vi "Calculate Batch Offset Values.vi"(8 "error in":errorcluster, 9 "Site Data":T2[](array[typedef]), 10 "Cal Runtime Cfg":T5, 11 "Config Data":T4(array[cluster])) -> (0 "error out":errorcluster, 1 "Data String":string[][](array[string]), 2 "Col Header String":string[](array[string]), 3 "All Items Pass?":bool, 4 "Limit Status":T1)   [LabVIEW 2020, in "GUCalibration2.lvlib"]
uses:
  GUCalibration2.lvlib
  Controls/Config Data Type.ctl
  Controls/Site Data Element.ctl
  Controls/Site Raw Data Element.ctl
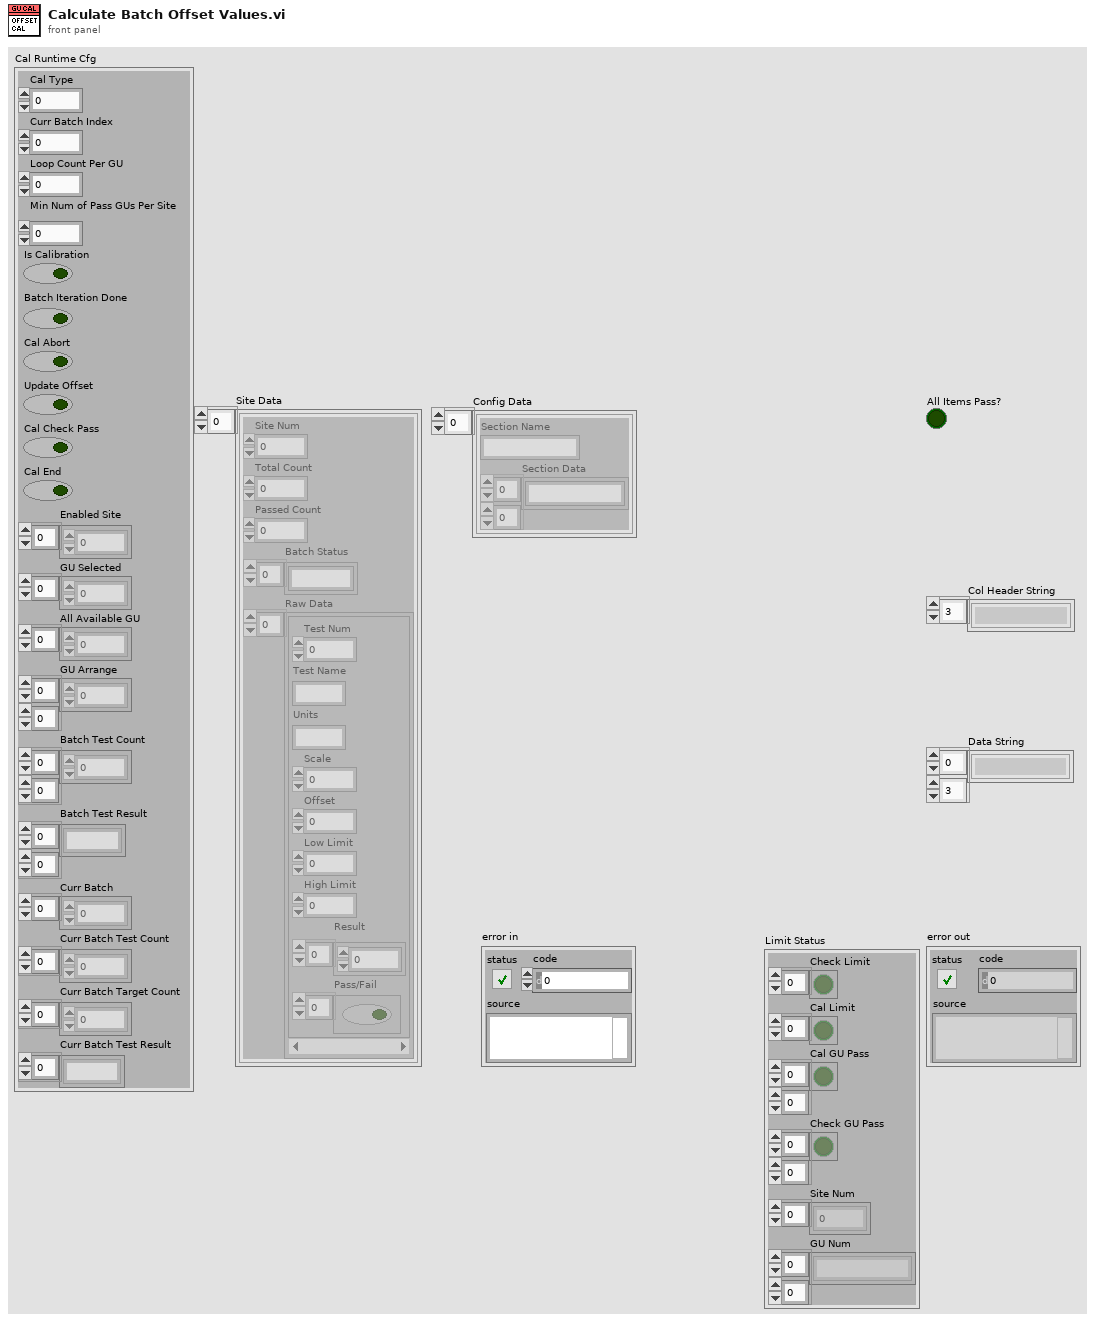
[diagram p1: front panel]
types:
  T1 = cluster{"Check Limit":bool[], "Cal Limit":bool[], "Cal GU Pass":bool[][], "Check GU Pass":bool[][], "Site Num":i32[], "GU Num":string[][]}
  T2 = typedef "GUCalibration2.lvlib/Site Data Element.ctl" = cluster{"Site Num":i32, "Total Count":i32, "Passed Count":i32, "Batch Status":string[], "Raw Data":T3[]}
  T3 = typedef "GUCalibration2.lvlib/Site Raw Data Element.ctl" = cluster{"Test Num":u32, "Test Name":string, "Units":string, "Scale":i8, "Offset":dbl, "Low Limit":dbl, "High Limit":dbl, "Result":dbl[], "Pass/Fail":bool[]}
  T4 = cluster{"Section Name":string, "Section Data":string[][]}[]
  T5 = typedef "GUCalibration2.lvlib/Config Data Type.ctl" = cluster{"Cal Type":i32, "Curr Batch Index":i32, "Loop Count Per GU":i32, "Min Num of Pass GUs Per Site":i32, "Is Calibration":bool, "Batch Iteration Done":bool, "Cal Abort":bool, "Update Offset":bool, "Cal Check Pass":bool, "Cal End":bool, "Enabled Site":i32[], "GU Selected":i32[], "All Available GU":i32[], "GU Arrange":i32[][], "Batch Test Count":i32[][], "Batch Test Result":string[][], "Curr Batch":i32[], "Curr Batch Test Count":i32[], "Curr Batch Target Count":i32[], "Curr Batch Test Result":string[]}
  T6 = cluster{"File Path":path, "Backup File Path":path, "Offset Data":cluster{"Section Name":string, "Section Data":string[][]}[]}
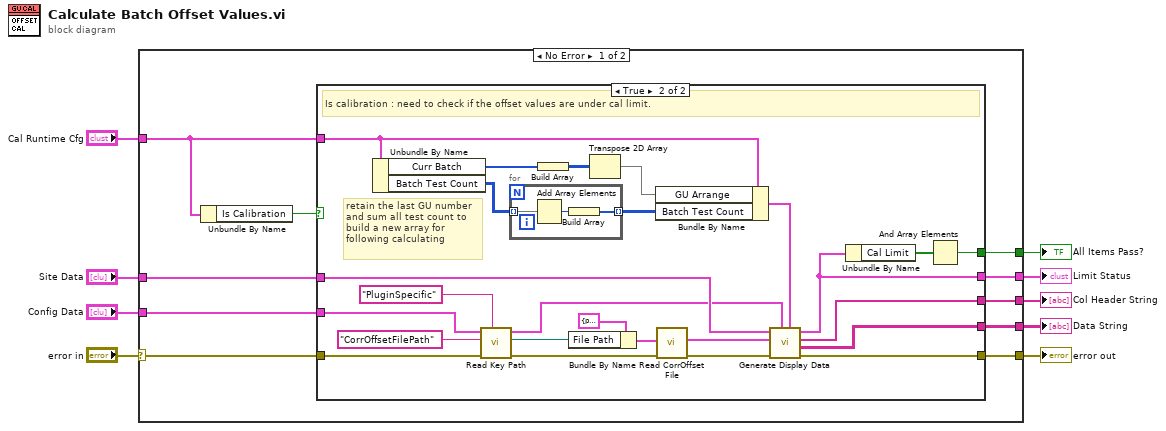
[diagram p0: block diagram]
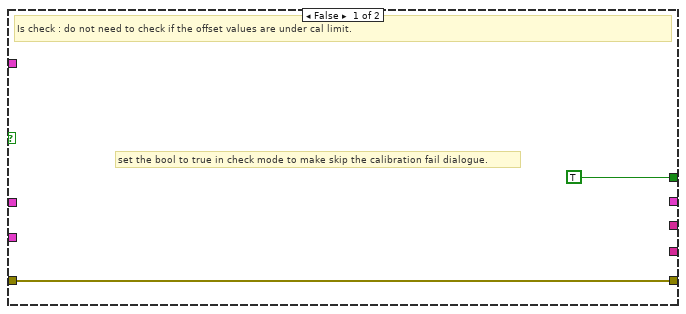
[diagram p2: hidden frame]
diagram:
  n1 = case shown="No Error" "error in" {
    selector: "error in" -> [w19 w50]
    tunnel: [w14 w50] -> w9
    tunnel: "Cal Runtime Cfg" -> [w15 _]
    tunnel: "Config Data" -> [w18 _]
    tunnel: "Site Data" -> [w17 _]
    tunnel: [w13 _] -> w4
    tunnel: [w12 _] -> w3
    tunnel: [w11 _] -> w2
    tunnel: [w10 _] -> w1
    frame No Error {
      n2 = Unbundle By Name(w15) -> ("Is Calibration"=w16:bool)
      n3 = case shown="True" w16 {
        tunnel: w19 -> [w21 w45]
        tunnel: w18 -> [_ w44]
        tunnel: w17 -> [_ w23]
        tunnel: w15 -> [_ w35]
        tunnel: [w21 w37] -> w14
        tunnel: [TRUE w25] -> w13
        tunnel: [_ w28] -> w12
        tunnel: [_ w27] -> w11
        tunnel: [_ w26] -> w10
        frame False {
          # "set the bool to true in check mode to make skip the calibration fail dialogue."
          # "Is check : do not need to check if the offset values are under cal limit."
        }
        frame True {
          # "retain the last GU number\nand sum all test count to \nbuild a new array for \nfollowing calculating"
          # "Is calibration : need to check if the offset values are under cal limit."
          n4 = Unbundle By Name(w35) -> ("Curr Batch"=w32:i32[], "Batch Test Count"=w31:i32[][])
          n5 = call "Read Key Path.vi"("Section Name"="PluginSpecific", "error in (no error)"=w45, "Key Names"="CorrOffsetFilePath" ("Section Name"), "Config Data"=w44) -> ("error out"=w43:errorcluster, "Key Value out"=w40:path, "Config Data dup"=w22:T4)  [unwired: 3 in, 2 out]
          n6 = for {
            tunnel: w31 -> [w49] mode=indexing
            tunnel: [w47] -> w30 mode=indexing
            n7 = Add Array Elements(numeric array=w49) -> (sum=w48:i32)
            n8 = Build Array(w48) -> (w47:i32[])
          }
          n9 = Build Array(w32) -> (w34:i32[][])
          n10 = Bundle By Name(cluster=T6 {"File Path"=path "", "Backup File Path"=path "", "Offset Data"=[]} ("CorrOffset File In"), "File Path"=w40) -> (w41:T6)
          n11 = Transpose 2D Array(2D array=w34) -> (transposed array=w33:i32[][])
          n12 = Bundle By Name(cluster=w35, "GU Arrange"=w33, "Batch Test Count"=w30) -> (w36:T5)
          n13 = call "Read CorrOffset File.vi"("error in"=w43, "CorrOffset File In"=w41) -> ("error out"=w24:errorcluster, "CorrOffset File Out"=w38:T6)  [unwired: 8 in]
          n14 = call "Generate Display Data.vi"("Cal Runtime Cfg"=w36, "Config Data"=w22, "error in"=w24, "CorrOffset File In"=w38, "Site Data"=w23) -> ("error out"=w37:errorcluster, "Data String"=w26:string[][], "Col Header String"=w27:string[], "Limit Status"=w28:T1)  [unwired: 2 in, 1 out]
          n15 = Unbundle By Name(w28) -> ("Cal Limit"=w29:bool[])
          n16 = And Array Elements(Boolean array=w29) -> (logical AND=w25:bool)
        }
      }
    }
    frame Error {
    }
  }
  "error out" <- w9
  "All Items Pass?" <- w4
  "Limit Status" <- w3
  "Col Header String" <- w2
  "Data String" <- w1
